vi "colourLUTcached.vi"(7 "rampMarkers":cluster{"value":dbl, "colour":u32}[](array[cluster])=[{"value"=100.0, "colour"=16711680}, {"value"=0.0, "colour"=16448250}, {"value"=-100.0, "colour"=16860}], 11 "value":dbl) -> (1 "values":dbl[](array[numeric]), 2 "colours":u32[](array[colorbox]), 3 "colour":u32(colorbox))   [LabVIEW 2021]
uses:
  150c2db4-2430-4a4b-9c53-d4e7b794cf9a.vi
  674f085b-e761-0c4b-8402-b427bb68fcd0.vi
  <vilib>/Analysis/1siggen.llb/Ramp Pattern by Samples.vi
  <vilib>/Comparison/Less/Less Functor/Less Functor.lvclass
  <vilib>/Analysis/NI_AALBase.lvlib
panel:
  in  "offLow":u32(colorbox)=50432
  in  "offHigh":u32(colorbox)=16699913
  in  "samples":i32=128
  out "ramper":dbl(ramp)
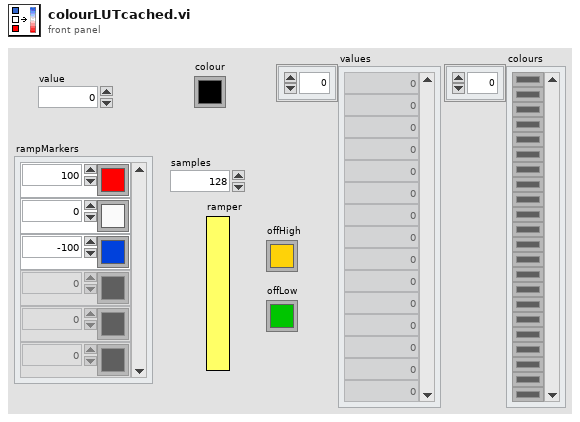
[diagram p1: front panel]
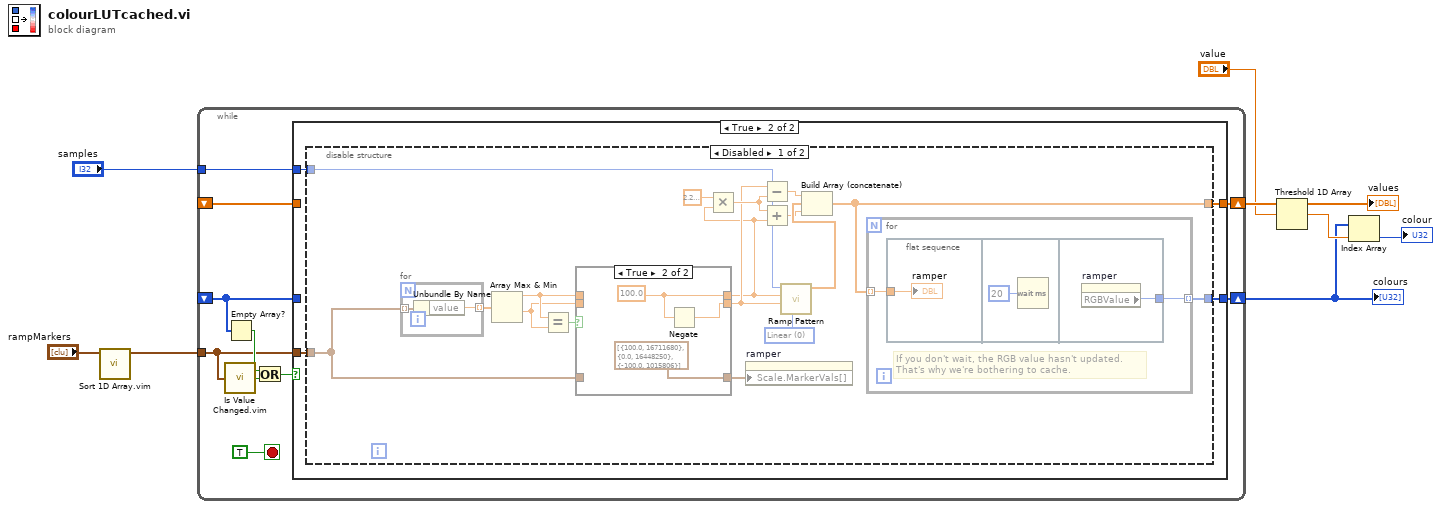
[diagram p0: block diagram]
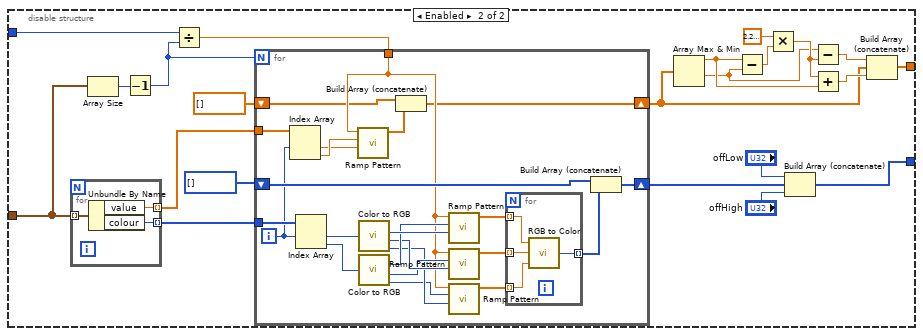
[diagram p4: hidden frame]
diagram:
  n1 = call "Sort 1D Array.vim"("unsorted array"="rampMarkers") -> ("sorted array"=w1:cluster{"value":dbl, "colour":u32}[])  [unwired: 10 in]
  n2 = while {
    tunnel: w1 -> [w10]
    shift-right: [w18] -> w8
    shift-left: _ -> [w15]
    shift-right: [w17] -> w6
    shift-left: _ -> [w14]
    tunnel: "samples" -> [w13]
    stop <- TRUE stop-if-true
    n3 = call "Is Value Changed.vim"("value"=w10) -> ("changed or first call?"=w9:bool)
    n4 = Empty Array?(array=w14) -> (empty?=w11:bool)
    n5 = Or(x=w11, y=w9) -> (x .or. y?=w12:bool)
    n6 = case shown="True" w12 {
      tunnel: [w20 w22] -> w18
      tunnel: [w19 w24] -> w17
      tunnel: w10 -> [_ w21]
      tunnel: w15 -> [w20 _]
      tunnel: w14 -> [w19 _]
      tunnel: w13 -> [_ w23]
      frame False {
      }
      frame True {
        n7 = disable-structure shown="Disabled" {
          disable-tunnel: [w39 w55] -> w24
          disable-tunnel: w23 -> [w37 w57]
          disable-tunnel: [w35 w56] -> w22
          disable-tunnel: w21 -> [w27 w58]
          frame Disabled {
            w41 = u16 0 items=["Linear", "Logarithmic"] ("type")
            n8 = for {
              tunnel: w27 -> [w49] mode=indexing
              tunnel: [w48] -> w38 mode=indexing
              n9 = Unbundle By Name(w49) -> ("value"=w48:dbl)
            }
            n10 = Array Max & Min(array=w38) -> (max value=w30:dbl, min value=w29:dbl)  [unwired: 2 out]
            n11 = Equal?(x=w30, y=w29) -> (x = y?=w31:bool)
            n12 = case shown="True" w31 {
              tunnel: [w44 w47] -> w25
              tunnel: [w43 w46] -> w28
              tunnel: w30 -> [w44 _]
              tunnel: w29 -> [w43 _]
              tunnel: w27 -> [w42 _]
              tunnel: [w42 cluster{"value":dbl, "colour":u32}[] [{"value"=100.0, "colour"=16711680}, {"value"=0.0, "colour"=16448250}, {"value"=-100.0, "colour"=1015806}] ("rampMarkers")] -> w26
              frame False {
              }
              frame True {
                w47 = 100.0 ("y")
                n13 = Negate(x=w47) -> (-x=w46:dbl)
              }
            }
            n14 = Multiply(x=2.220446049250313e-16, y=w25) -> (x*y=w32:dbl)
            n15 = property on="ramper" class="ColRmp (strict)"("Scale.MarkerVals[]"=w26) -> ()  [unwired: 2 in, 2 out]
            n16 = Subtract(x=w28, y=w32) -> (x-y=w34:dbl)
            n17 = Add(x=w32, y=w25) -> (x+y=w33:dbl)
            n18 = call-poly <vilib>:"Ramp Pattern.vi"("type"=w41, "start"=w28, "end"=w25, "samples"=w37) -> ("Ramp Pattern"=w40:dbl[])  [unwired: 6 in, 1 out]
            n19 = Build Array (concatenate)(w34, w40, w33) -> (w35:dbl[])
            n20 = for {
              tunnel: w35 -> [w51] mode=indexing
              tunnel: [w50] -> w39 mode=indexing
              # "If you don't wait, the RGB value hasn't updated.\nThat's why we're bothering to cache."
              n21 = flat-sequence {
                tunnel: w51 -> [w52]
                tunnel: [w54] -> w50
                frame #0 {
                  "ramper" <- w52
                }
                frame #1 {
                  n22 = Wait (ms)(milliseconds to wait=u32 20) -> ()  [unwired: 1 out]
                }
                frame #2 {
                  n23 = property on="ramper" class="ColRmp (strict)"() -> ("RGBValue"=w54:u32)  [unwired: 2 in, 2 out]
                }
              }
            }
          }
          frame Enabled {
            n24 = for {
              tunnel: w58 -> [w79] mode=indexing
              tunnel: [w78] -> w76 mode=indexing
              tunnel: [w77] -> w71 mode=indexing
              n25 = Unbundle By Name(w79) -> ("value"=w77:dbl, "colour"=w78:u32)
            }
            n26 = Array Size(array=w58) -> (size(s)=w74:i32)
            n27 = Decrement(x=w74) -> (x-1=w73:i32)
            n28 = Divide(x=w57, y=w73) -> (x/y=w72:dbl)
            n29 = for {
              N: w73 -> [_]
              shift-right: [w99] -> w75
              shift-left: u32[] [] -> [w100]
              tunnel: w76 -> [w96]
              tunnel: w72 -> [w85]
              tunnel: w71 -> [w87]
              shift-right: [w82] -> w67
              shift-left: dbl[] [] -> [w83]
              i -> [w86]
              n30 = Index Array(array=w87, index #1=w86) -> (element #1=w80:dbl, element #2=w81:dbl)  [unwired: 1 in]
              n31 = Index Array(array=w96, index #1=w86) -> (element #1=w95:u32, element #2=w94:u32)  [unwired: 1 in]
              n32 = call-poly <vilib>:"Ramp Pattern.vi"("start"=w80, "end"=w81, "samples"=w85) -> ("Ramp Pattern"=w84:dbl[])  [unwired: 7 in, 1 out]
              n33 = call <vilib>:"Color to RGB.vi"("Color"=w95) -> ("R"=w93:u8, "G"=w91:u8, "B"=w89:u8)  [unwired: 1 out]
              n34 = call <vilib>:"Color to RGB.vi"("Color"=w94) -> ("R"=w92:u8, "G"=w90:u8, "B"=w88:u8)  [unwired: 1 out]
              n35 = Build Array (concatenate)(w83, w84) -> (w82:dbl[])
              n36 = call-poly <vilib>:"Ramp Pattern.vi"("start"=w93, "end"=w92, "samples"=w85) -> ("Ramp Pattern"=w102:dbl[])  [unwired: 7 in, 1 out]
              n37 = call-poly <vilib>:"Ramp Pattern.vi"("start"=w91, "end"=w90, "samples"=w85) -> ("Ramp Pattern"=w98:dbl[])  [unwired: 7 in, 1 out]
              n38 = call-poly <vilib>:"Ramp Pattern.vi"("start"=w89, "end"=w88, "samples"=w85) -> ("Ramp Pattern"=w97:dbl[])  [unwired: 7 in, 1 out]
              n39 = for {
                tunnel: w102 -> [w105] mode=indexing
                tunnel: w98 -> [w106] mode=indexing
                tunnel: w97 -> [w104] mode=indexing
                tunnel: [w103] -> w101 mode=indexing
                n40 = call <vilib>:"RGB to Color.vi"("B"=w104, "G"=w106, "R"=w105) -> ("Color"=w103:u32)
              }
              n41 = Build Array (concatenate)(w100, w101) -> (w99:u32[])
            }
            n42 = Array Max & Min(array=w67) -> (max value=w66:dbl, min value=w65:dbl)  [unwired: 2 out]
            n43 = Subtract(x=w66, y=w65) -> (x-y=w64:dbl)
            n44 = Multiply(x=2.220446049250313e-16, y=w64) -> (x*y=w68:dbl)
            n45 = Build Array (concatenate)("offLow", w75, "offHigh") -> (w55:u32[])
            n46 = Subtract(x=w65, y=w68) -> (x-y=w70:dbl)
            n47 = Add(x=w68, y=w66) -> (x+y=w69:dbl)
            n48 = Build Array (concatenate)(w70, w67, w69) -> (w56:dbl[])
          }
        }
      }
    }
  }
  "values" <- w8
  "colours" <- w6
  n49 = Threshold 1D Array(2:"value", 3:w8) -> (0:w7:dbl)  [unwired: 1 in]
  n50 = Index Array(array=w6, index=w7) -> (element=→"colour":u32)
